vi "setup complete.vi"() -> ()   [LabVIEW 2014]
panel:
  in  "?":bool
  out "메시지":string
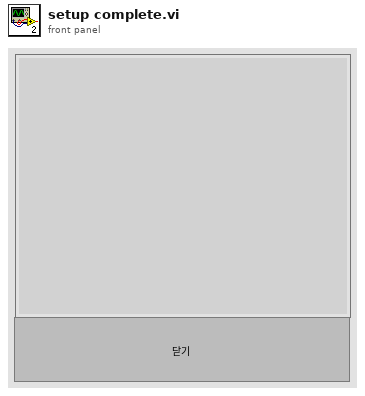
[diagram p1: front panel]
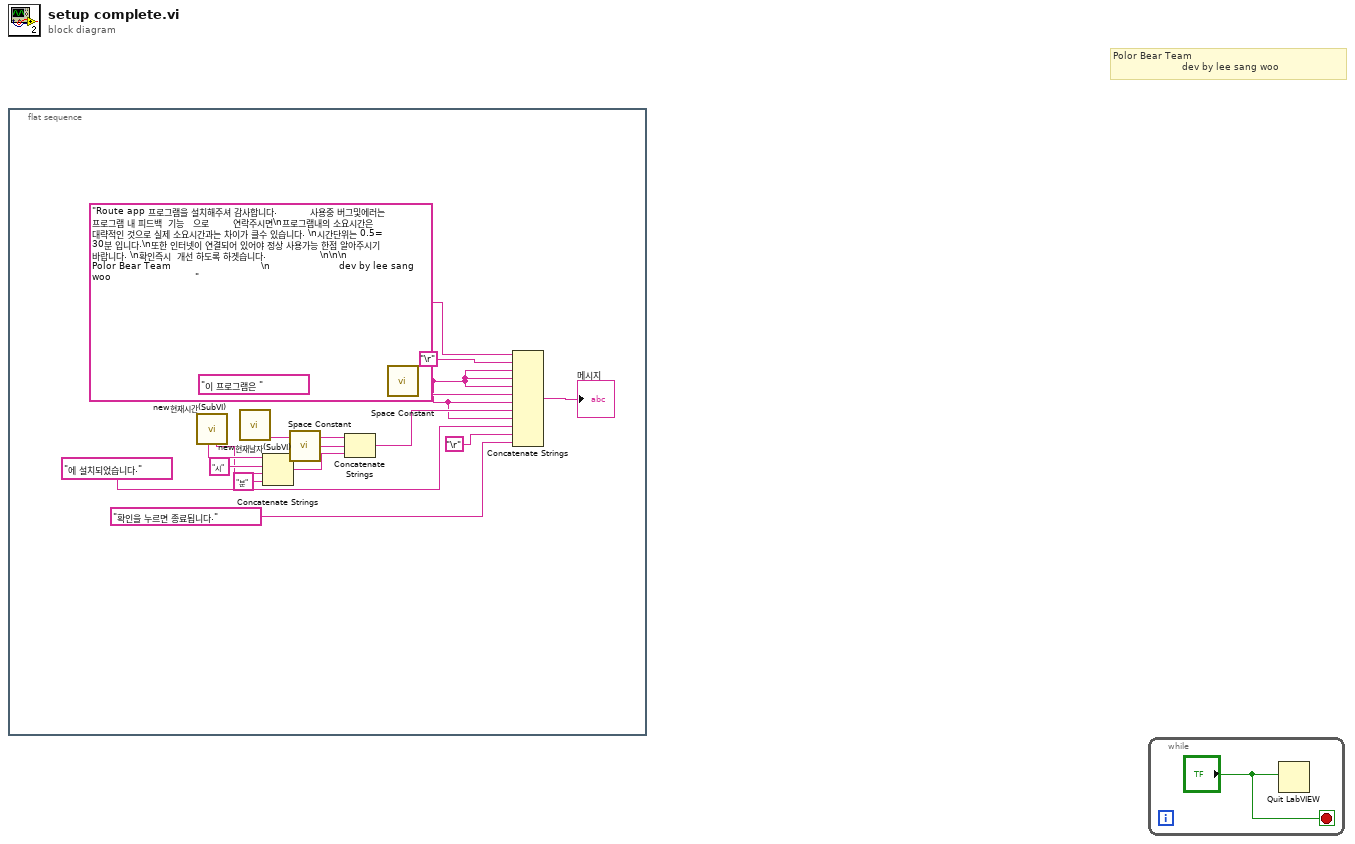
[diagram p0: block diagram]
diagram:
  # "Polor Bear Team                              \n                       dev by lee sang woo"
  n1 = flat-sequence {
    frame #0 {
      n2 = call "new현재시간(SubVI).vi"() -> ("분 문자열"=w14:string, "시 문자열"=w16:string)  [unwired: 3 in, 7 out]
      n3 = call "new현재날자(SubVI).vi"() -> ("월,일 을 문자열로"=w10:string)  [unwired: 5 in, 6 out]
      n4 = Concatenate Strings(w16, "시", w14, "분" ("문자열")) -> (w12:string)
      n5 = call <vilib>:"Space Constant.vi"() -> ("String"=w11:string)
      n6 = Concatenate Strings(w10, w11, w12) -> (w6:string)
      n7 = call <vilib>:"Space Constant.vi"() -> ("String"=w5:string)
      n8 = Concatenate Strings("Route app 프로그램을 설치해주셔 감사합니다.           사용중 버그및에러는 프로그램 내 피드백  기능   으로        연락주시면\n프로그램내의 소요시간은 대략적인 것으로 실제 소요시간과는 차이가 클수 있습니다. \n시간단위는 0.5= 30분 입니다.\n또한 인터넷이 연결되어 있어야 정상 사용가능 한점 알아주시기 바랍니다. \n확인즉시  개선 하도록 하겟습니다.                  \n\n\n                           Polor Bear Team                              \n                       dev by lee sang woo                            " ("Message"), "\r", w5, w5, w5, "이 프로그램은 ", w5, w6, w5, "에 설치되었습니다.", "\r", "확인을 누르면 종료됩니다.") -> (→"메시지":string)
    }
  }
  n9 = while {
    stop <- "?" stop-if-true
    n10 = Quit LabVIEW(quit? (T)="?") -> ()
  }
